vi "Change Setting.vi"(8 "error in (no error)":errorcluster, 10 "Change setting mode":T1=enum."Next", 11 "Device-Thru in":refnum<class "Thru.lvclass">) -> (0 "error out":errorcluster, 1 "Changes":cluster{"Name":string, "Value":string}[](array[cluster]), 2 "Last setting":bool, 3 "Device-Thru out":refnum<class "Thru.lvclass">)   [LabVIEW 2020, in "Thru.lvclass"]
uses:
  Thru.lvclass
  Controls/Change setting mode enum.ctl
  PIC-device/PIC-Device.lvclass
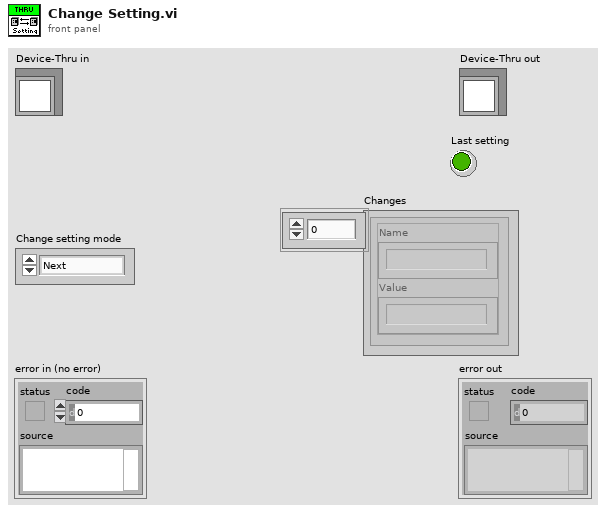
[diagram p1: front panel]
types:
  T1 = typedef "PIC-Device.lvclass/Change setting mode enum.ctl" = enum16{"Init", "Next", "Reset"}
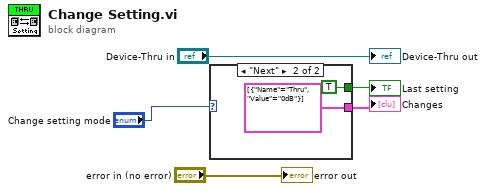
[diagram p0: block diagram]
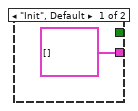
[diagram p2: hidden frame]
diagram:
  n1 = case shown="\"Next\"" "Change setting mode" {
    tunnel: [cluster{"Name":string, "Value":string}[] [] ("Changes") cluster{"Name":string, "Value":string}[] [{"Name"="Thru", "Value"="0dB"}] ("Changes")] -> w3
    tunnel: [_ TRUE] -> w1
    frame "Init", Default {
    }
    frame "Next" {
    }
  }
  "Changes" <- w3
  "Last setting" <- w1
  "error out" <- "error in (no error)"
  "Device-Thru out" <- "Device-Thru in"
